vi "Change Input DT.vi"(6 "Variant":variant, 8 "error in (no error)":errorcluster, 9 "old values":string[][](array[string]), 10 "object ref in":T2, 11 "Cluster":T3) -> (0 "error out":errorcluster)   [LabVIEW 2013, in "Scaling editor node.lvclass"]
uses:
  Scaling editor node.lvclass
  <vilib>/NI/DCAF Table API/Table Manager/Cell Change.ctl
  <vilib>/NI/DCAF Table API/Table Manager/object ref.ctl
  <vilib>/NI/DCAF/Tag Editor Core/Configuration Editor/Classes/Engine Parent/Engine Parent Editor Node.lvclass
  <vilib>/NI/DCAF/Tag Editor Core/Configuration Editor/Classes/Module editor node/module editor node.lvclass
  module/configuration/controls/scale data types.ctl
  module/configuration/Scaling configuration.lvclass
  Scaling editor node.lvclass/Scaling editor node.ctl
  <vilib>/NI/DCAF Table API/Table Manager.lvlib
  <vilib>/NI/DCAF Table API/Table Manager/Table Manager.lvclass
panel:
  in  "dt":T1
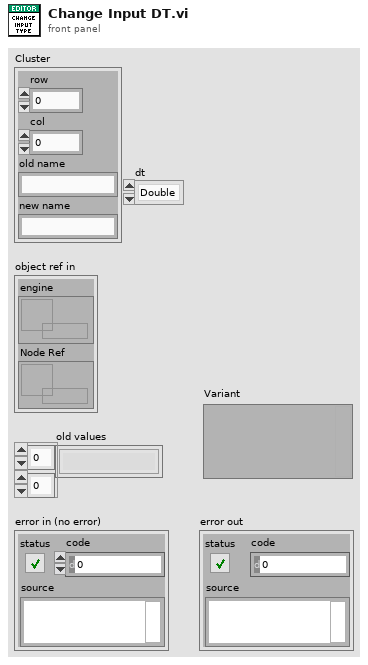
[diagram p1: front panel]
types:
  T1 = typedef "Scaling configuration.lvclass/scale data types.ctl" = enum16{"Double", "Single", "I64", "I32", "I16", "I8", "U64", "U32", "U16", "U8"}
  T2 = typedef "Table Manager.lvlib/Table Manager.lvclass/object ref.ctl" = cluster{"engine":refnum<data-value>, "Node Ref":refnum<data-value>}
  T3 = typedef "Table Manager.lvlib/Cell Change.ctl" = cluster{"row":i32, "col":i32, "old name":string, "new name":string}
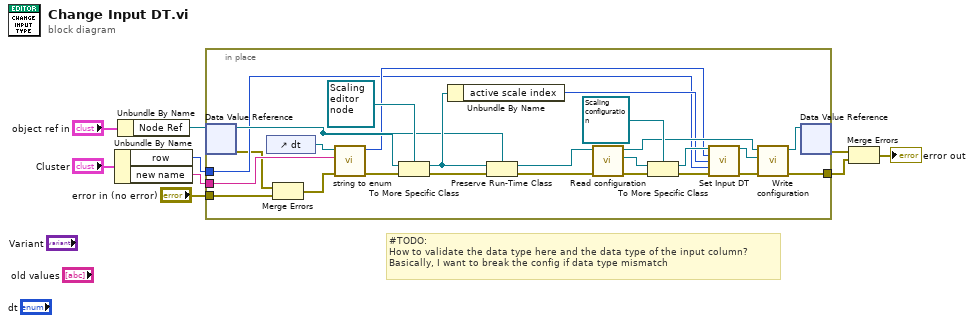
[diagram p0: block diagram]
diagram:
  # "#TODO:\nHow to validate the data type here and the data type of the input column?\nBasically, I want to break the config if data type mismatch"
  n1 = Unbundle By Name("Cluster") -> ("row"=w8:i32, "new name"=w2:string)
  n2 = Unbundle By Name("object ref in") -> ("Node Ref"=w9:refnum<data-value>)
  n3 = in-place {
    in-place-border: w8 -> [w13]
    in-place-border: [w25] -> w4
    in-place-border: w2 -> [w16]
    in-place-border: "error in (no error)" -> [w11]
    n4 = in-place-dvr #1(w9) -> (w24:refnum<class "module editor node.lvclass">, w12:errorcluster)
    n5 = control-ref of="dt"() -> (w17:refnum<vi>)
    n6 = Merge Errors(w12, w11) -> (w10:errorcluster)
    n7 = call <vilib>:"string to enum.vi"("error in"=w10, "String"=w16, "Enum"=w17) -> ("error out"=w18:errorcluster, "Value"=w15:i32)  [unwired: 7 in]
    n8 = To More Specific Class(target class=refnum<class "Scaling editor node.lvclass"> refnum ("Scaling editor node"), reference=w24, error in=w18) -> (specific class reference=w30:refnum<class "Scaling editor node.lvclass">, error out=w23:errorcluster)
    n9 = Unbundle By Name(w30) -> ("active scale index"=w14:i32)
    n10 = Preserve Run-Time Class(object in=w30, error in=w23, 2:w24) -> (object out=w29:refnum<class "module editor node.lvclass">, error out=w28:errorcluster)
    n11 = call-dynamic "Read configuration.vi"("error in"=w28, "NISE_CEF_serializable node in"=w29) -> ("error out"=w27:errorcluster, "configuration"=w32:refnum<class "NISE_CEF_serializable configuration.lvclass">, "NISE_CEF_serializable node out"=w26:refnum<class "module editor node.lvclass">)  [unwired: 7 in]
    n12 = To More Specific Class(target class=refnum<class "Scaling configuration.lvclass"> refnum ("Scaling configuration"), reference=w32, error in=w27) -> (specific class reference=w19:refnum<class "Scaling configuration.lvclass">, error out=w20:errorcluster)
    n13 = call "Set Input DT.vi"("Scaling configuration in"=w19, "Scale Data Type"=w15, "Scale Index"=w14, "Mapping Index"=w13, "error in (no error)"=w20) -> ("Scaling configuration out"=w22:refnum<class "Scaling configuration.lvclass">, "error out"=w21:errorcluster)  [unwired: 9 in]
    n14 = call-dynamic "Write configuration.vi"("error in"=w21, "configuration"=w22, "NISE_CEF_serializable node in"=w26) -> ("error out"=w25:errorcluster, "NISE_CEF_serializable node out"=w34:refnum<class "module editor node.lvclass">)  [unwired: 7 in]
    n15 = in-place-dvr #1(w34) -> (w5:errorcluster)  [unwired: 1 out]
  }
  n16 = Merge Errors(w5, w4) -> (→"error out":errorcluster)
